vi "Dictionary Get Value__ogtk.vi"(7 "lock dictionary if key is found? (FALSE)":bool, 8 "error in":errorcluster, 10 "key":variant, 11 "dictionary":T1) -> (0 "error out":errorcluster, 1 "found?":bool, 2 "value":variant, 3 "dictionary out":T1)   [LabVIEW 2020]
doc: "Returns the value associated with key, if it exists. If the dictionary has the specified key, then found? will be TRUE.\n\n<B>lock dictionary if key is found?</B> will lock the dictionary (only if the key is found), preventing dictionary modifications until it is unlocked. Locking a dictionary is useful when the values of keys store compound data, which might be modified in multiple locations. The dictionary may be unlocked using the <B>unlock dictionary</B> input of the <B>Update Dictionary</B> function."
uses:
  <userlib>/_OpenG.lib/dictionary/dictionary.llb/Dictionary Object RefNum__ogtk.ctl
  <userlib>/_OpenG.lib/dictionary/dictionary.llb/Dictionary Object RefNum - Enum__ogtk.ctl
panel:
  # "Dictionary Get Value.vi\n\nReturns the value associated with key, if it exists.\n\nPlease visit http://www.OpenG.org to learn about the\nOpen Source LabVIEW software movement.\n\nNOTICE -- YOU MUST LEAVE THIS NOTICE IN PLACE.  PER THE TERMS OF THE LICENSE BELOW, YOU MAY SUBLICENSE THIS SOFTWARE \nIN ANY WAY THAT DOES NOT CONFLICT WITH THIS LICENSE.\n\n### BSD License (http://www.opensource.org/licenses/bsd-license.php) Begin ###\n \nCopyright (c) 2005, Jim Kring <jim@jimkring.com>\n\nAll rights reserved.\n\nRedistribution and use in source and binary forms, with or without modification, are permitted provided that the following conditions are met:\n\n    * Redistributions of source code must retain the above copyright notice, this list of conditions and the following disclaimer.\n    * Redistributions in binary form must reproduce the above copyright notice, this list of conditions and the following disclaimer in the \n       documentation and/or other materials provided with the distribution.\n    * Neither the name of SciWare, James Kring, Inc., nor the names of its contributors may be used to endorse or promote products derived \n       from this software without specific prior written permission.\n\nTHIS SOFTWARE IS PROVIDED BY THE COPYRIGHT HOLDERS AND CONTRIBUTORS \"AS IS\" AND ANY EXPRESS OR IMPLIED WARRANTIES, \nINCLUDING, BUT NOT LIMITED TO, THE IMPLIED WARRANTIES OF MERCHANTABILITY AND FITNESS FOR A PARTICULAR PURPOSE ARE \nDISCLAIMED. IN NO EVENT SHALL THE COPYRIGHT OWNER OR CONTRIBUTORS BE LIABLE FOR ANY DIRECT, INDIRECT, INCIDENTAL,\n SPECIAL, EXEMPLARY, OR CONSEQUENTIAL DAMAGES (INCLUDING, BUT NOT LIMITED TO, PROCUREMENT OF SUBSTITUTE GOODS OR \nSERVICES; LOSS OF USE, DATA, OR PROFITS; OR BUSINESS INTERRUPTION) HOWEVER CAUSED AND ON ANY THEORY OF LIABILITY, \nWHETHER IN CONTRACT, STRICT LIABILITY, OR TORT (INCLUDING NEGLIGENCE OR OTHERWISE) ARISING IN ANY WAY OUT OF THE USE \nOF THIS SOFTWARE, EVEN IF ADVISED OF THE POSSIBILITY OF SUCH DAMAGE.\n\n### BSD License End ###"
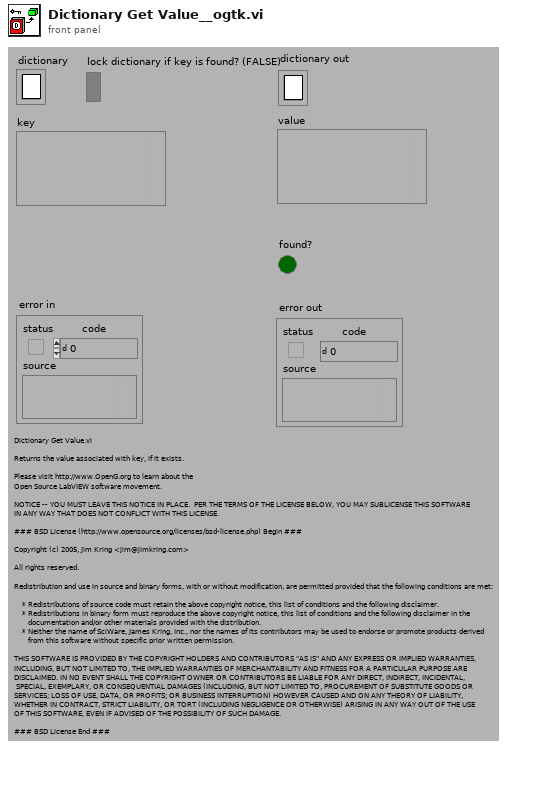
[diagram p1: front panel]
types:
  T1 = typedef "Dictionary Object RefNum__ogtk.ctl" = refnum<k1>
  T2 = typedef "Dictionary Data__ogtk.ctl" = cluster{"keys":variant[], "values":variant[]}
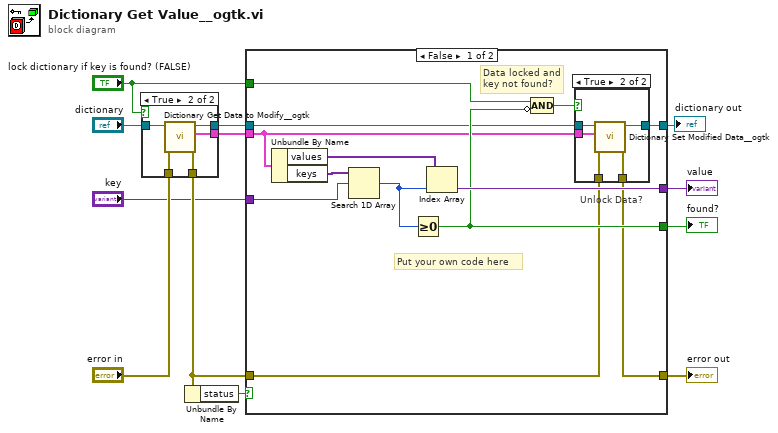
[diagram p0: block diagram]
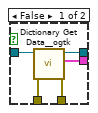
[diagram p2: hidden frame]
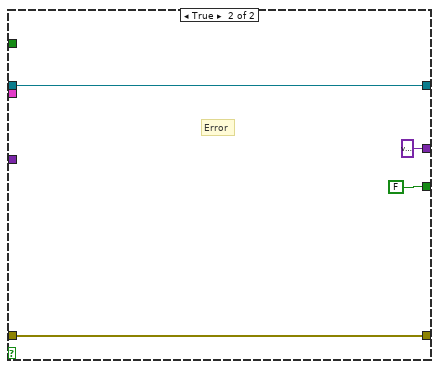
[diagram p4: hidden frame]
diagram:
  n1 = case shown="True" "lock dictionary if key is found? (FALSE)" {
    tunnel: [w17 w20] -> w10
    tunnel: "error in" -> [w16 w22]
    tunnel: [w15 w21] -> w8
    tunnel: [w14 w18] -> w2
    tunnel: "dictionary" -> [w13 w19]
    frame False {
      n2 = call <userlib>:"Dictionary Get Data__ogtk.vi"("error in (no error)"=w16, "Object RefNum"=w13) -> ("error out"=w15:errorcluster, "Data out"=w17:T2, "Dup Object RefNum"=w14:T1)  [unwired: 7 in]
    }
    frame True {
      n3 = call <userlib>:"Dictionary Get Data to Modify__ogtk.vi"("error in (no error)"=w22, "Object RefNum"=w19) -> ("error out"=w21:errorcluster, "Data out"=w20:T2, "Dup Object RefNum"=w18:T1)  [unwired: 6 in, 1 out]
    }
  }
  n4 = Unbundle By Name(w8) -> ("status"=w12:bool)
  n5 = case shown="False" w12 {
    tunnel: w8 -> [w25 w46]
    tunnel: [w24 w46] -> w11
    tunnel: w10 -> [w28 _]
    tunnel: "key" -> [w34 _]
    tunnel: [w30 FALSE] -> w5
    tunnel: [w31 variant ("Variant")] -> w4
    tunnel: "lock dictionary if key is found? (FALSE)" -> [w29 _]
    tunnel: w2 -> [w26 w43]
    tunnel: [w23 w43] -> w1
    frame False {
      # "Data locked and key not found?"
      # "Put your own code here"
      n6 = Unbundle By Name(w28) -> ("values"=w32:variant[], "keys"=w35:variant[])
      n7 = Search 1D Array(1D array=w35, element=w34) -> (index of element=w33:i32)  [unwired: 1 in]
      n8 = Greater Or Equal To 0?(x=w33) -> (x >= 0?=w30:bool)
      n9 = Index Array(array=w32, index=w33) -> (element=w31:variant)
      n10 = Compound Arithmetic op=AND(w29, invert w30) -> (w27:bool)
      n11 = case "Unlock Data?" shown="True" w27 {
        tunnel: w28 -> [_ w42]
        tunnel: w26 -> [w36 w41]
        tunnel: w25 -> [w37 w40]
        tunnel: [w37 w39] -> w24
        tunnel: [w36 w38] -> w23
        frame False {
        }
        frame True {
          n12 = call <userlib>:"Dictionary Set Modified Data__ogtk.vi"("error in (no error)"=w40, "Data in"=w42, "Object RefNum"=w41) -> ("error out"=w39:errorcluster, "dup Object RefNum"=w38:T1)  [unwired: 7 in]
        }
      }
    }
    frame True {
      # "Error"
    }
  }
  "error out" <- w11
  "dictionary out" <- w1
  "value" <- w4
  "found?" <- w5
